vi "readBatteryVoltage.vi"(8 "error in (no error)":errorcluster, 11 "Refnum in":T1) -> (0 "error out":errorcluster, 2 "Battery Voltage (V)":dbl, 3 "Refnum out":T1)   [LabVIEW 2011]
uses:
  SPI_TEST_REF.ctl
  <vilib>/Utility/error.llb/Error Cluster From Error Code.vi
  <vilib>/rvi/errors/niLvFpgaAdjustHostInterfaceError.vi
  <vilib>/rvi/interface/nirviReadWriteControl/nirviReadWriteControl.xnode
  FPGA Bitfiles/SailBot_FPGATarget3_VBattSenseSPITes_222C18A6.lvbitx
  1,3 A-Competition Platform/1,3 A Code/FPGA/VBattSense SPI Test.vi
  NiFpgaLv.dll
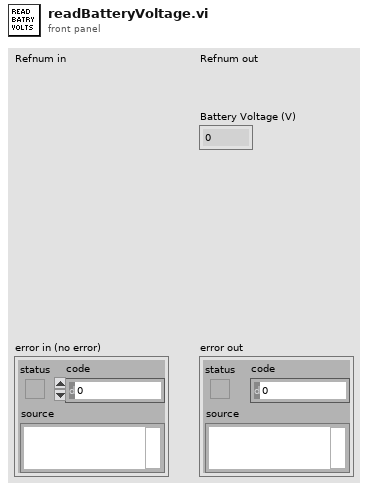
[diagram p1: front panel]
types:
  T1 = typedef "SPI_TEST_REF.ctl" = refnum<k20>
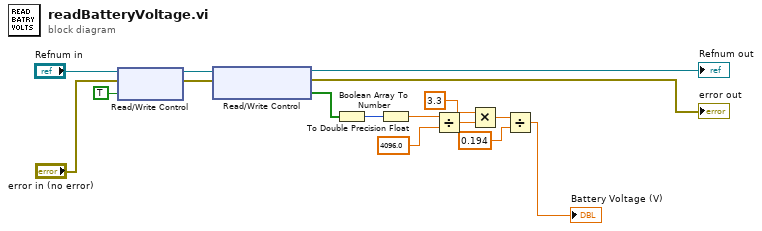
[diagram p0: block diagram]
diagram:
  n1 = xnode "Read/Write Control"("FPGA VI Reference In"="Refnum in", "error in"="error in (no error)", "SPI_Read"=TRUE) -> ("FPGA VI Reference Out"=w6:T1, "error out"=w7:errorcluster)
  n2 = xnode "Read/Write Control"("FPGA VI Reference In"=w6, "error in"=w7) -> ("FPGA VI Reference Out"=→"Refnum out":T1, "error out"=→"error out":errorcluster, "Battery Voltage"=w16:bool[])
  n3 = Boolean Array To Number(Boolean array=w16) -> (number=w2:u16)
  n4 = To Double Precision Float(number=w2) -> (double precision float=w1:dbl)
  n5 = Divide(x=w1, y=4096.0) -> (x/y=w11:dbl)
  n6 = Multiply(x=3.3, y=w11) -> (x*y=w13:dbl)
  n7 = Divide(x=w13, y=0.194) -> (x/y=→"Battery Voltage (V)":dbl)
